vi "Init.vi"(7 "I2C #":T1=-1, 8 "error in (no error)":errorcluster, 10 "Session In":refnum<class "Session.lvclass">) -> (0 "error out":errorcluster, 3 "I2C_0-20mA(GP8313) Out":refnum<class "I2C_0-20mA(GP8313).lvclass">)   [LabVIEW 2020, in "CTI-Peripheral.lvlib" / "I2C_0-20mA(GP8313).lvclass"]
uses:
  I2C_0-20mA(GP8313).lvclass
  CTI/Session/Session.lvclass
  CTI/I2C Number.ctl
  CTI/I2C Address.ctl
  CTI/I2C Connection/I2C Connection.lvclass/I2C Connection.ctl
  I2C_0-20mA(GP8313).lvclass/I2C_0-20mA(GP8313).ctl
  CTI/I2C Connection/I2C Connection.lvclass
  CTI/CTI.lvlib
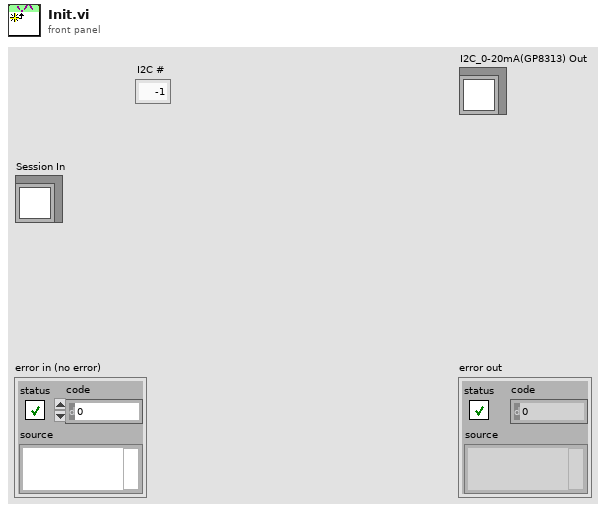
[diagram p1: front panel]
types:
  T1 = typedef "CTI.lvlib/I2C Number.ctl" = i8
  T2 = typedef "CTI.lvlib/I2C Address.ctl" = u8
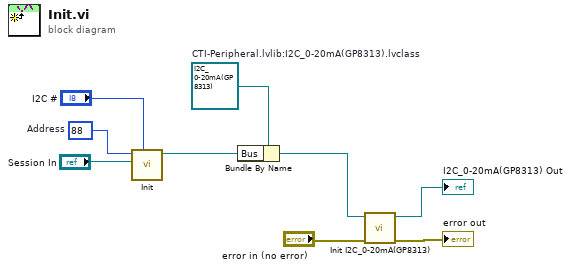
[diagram p0: block diagram]
diagram:
  w5 = refnum<class "I2C_0-20mA(GP8313).lvclass"> refnum  # CTI-Peripheral.lvlib:I2C_0-20mA(GP8313).lvclass
  w6 = T2 88  # Address
  n1 = call "Init.vi"("I2C #"="I2C #", "Session"="Session In", "Address"=w6) -> ("I2C Connection"=w9:refnum<class "I2C Connection.lvclass">)  [unwired: 7 in, 1 out]
  n2 = Bundle By Name(cluster=w5, "Bus"=w9) -> (w2:refnum<class "I2C_0-20mA(GP8313).lvclass">)
  n3 = call "Init I2C_0-20mA(GP8313).vi"("error in (no error)"="error in (no error)", "I2C_0-20mA(GP8212) in"=w2) -> ("error out"=→"error out":errorcluster, "I2C_0-20mA(GP8212) out"=→"I2C_0-20mA(GP8313) Out":refnum<class "I2C_0-20mA(GP8313).lvclass">)  [unwired: 8 in]
